vi "Launch Listener.vi"(8 "error in (no error)":errorcluster, 11 "Server Controller in":refnum<class "Server Controller.lvclass">) -> (0 "error out":errorcluster, 3 "Server Controller out":refnum<class "Server Controller.lvclass">)   [LabVIEW 2016, in "Server Controller.lvlib" / "Server Controller.lvclass"]
uses:
  Server Controller.lvclass
  C:/Program Files (x86)/National Instruments/LabVIEW 2016/vi.lib/ActorFramework/Actor/Actor.lvclass
  Listener/ServerListener.lvclass
  Server Controller.lvclass/Server Controller.ctl
  <vilib>/ActorFramework/Actor/Actor.lvclass/Actor.ctl
  <vilib>/ActorFramework/Message Enqueuer/Message Enqueuer.lvclass/Message Enqueuer.ctl
  Listener/ServerListener.lvclass/ServerListener.ctl
  <vilib>/ActorFramework/Message Enqueuer/Init from Existing Queue.vi
  <vilib>/ActorFramework/Message Enqueuer/Message Enqueuer.lvclass
  <vilib>/ActorFramework/Actor/Actor.lvclass
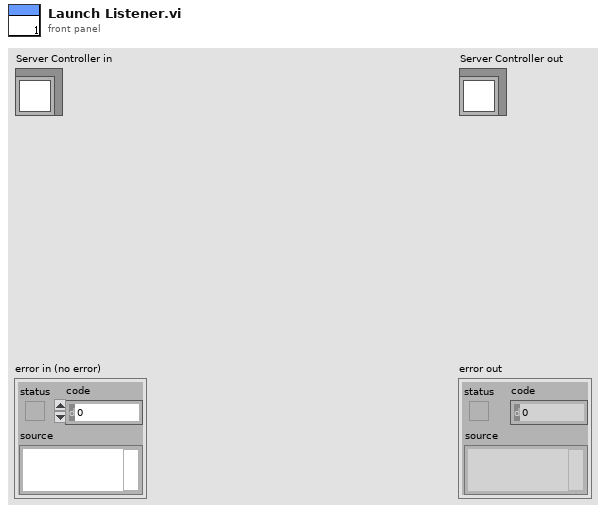
[diagram p1: front panel]
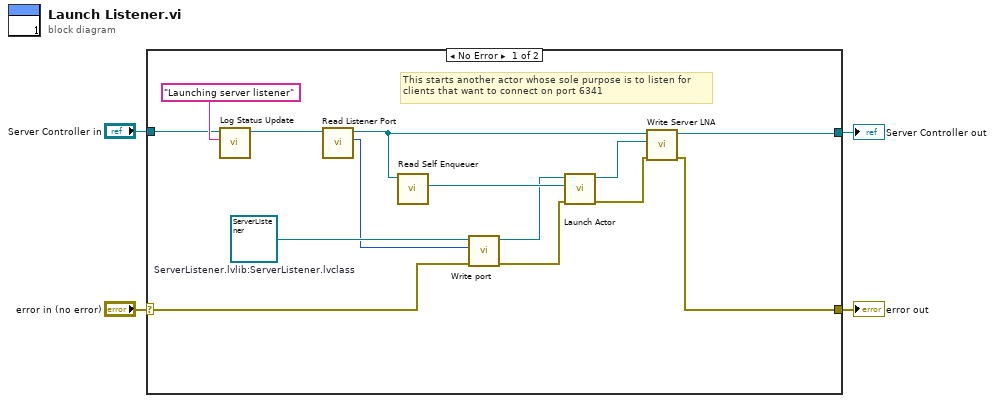
[diagram p0: block diagram]
diagram:
  n1 = case shown="No Error" "error in (no error)" {
    selector: "error in (no error)" -> [w12 w20]
    tunnel: [w16 w20] -> w3
    tunnel: [w8 w19] -> w1
    tunnel: "Server Controller in" -> [w9 w19]
    frame No Error {
      w14 = refnum<class "ServerListener.lvclass"> refnum  # ServerListener.lvlib:ServerListener.lvclass
      # "This starts another actor whose sole purpose is to listen for\nclients that want to connect on port 6341"
      n2 = call-dynamic "Log Status Update.vi"("String"="Launching server listener", "Controller in"=w9) -> ("Controller out"=w7:refnum<class "Server Controller.lvclass">)  [unwired: 8 in, 1 out]
      n3 = call "Read Listener Port.vi"("Server Controller in"=w7) -> ("Listener Port"=w5:u16, "Server Controller out"=w6:refnum<class "Server Controller.lvclass">)  [unwired: 8 in, 1 out]
      n4 = call <vilib>:"Read Self Enqueuer.vi"("Actor"=w6) -> ("Self Enqueuer"=w17:refnum<class "Message Enqueuer.lvclass">)  [unwired: 10 in]
      n5 = call "Write port.vi"("error in (no error)"=w12, "port"=w5, "ServerListener in"=w14) -> ("error out"=w11:errorcluster, "ServerListener out"=w13:refnum<class "ServerListener.lvclass">)  [unwired: 7 in]
      n6 = call <vilib>:"Launch Actor.vi"("error in (no error)"=w11, "Actor-to-Caller Enqueuer"=w17, "Actor"=w13) -> ("error out"=w15:errorcluster, "Caller-To-Actor Enqueuer"=w18:refnum<class "Message Enqueuer.lvclass">)  [unwired: 7 in]
      n7 = call "Write Server LNA.vi"("error in (no error)"=w15, "Actor Framework:Message Enqueuer"=w18, "Server Controller in"=w6) -> ("error out"=w16:errorcluster, "Server Controller out"=w8:refnum<class "Server Controller.lvclass">)  [unwired: 7 in]
    }
    frame Error {
    }
  }
  "error out" <- w3
  "Server Controller out" <- w1
